vi "PH_PILS.Dialog EO.vi"() -> (0 "EO Comment":string)   [LabVIEW 2014, in "PH_PILS.lvlib"]
doc: "This VI creates the entry for the logbook in case of emergency off and writes it to the Logfile D:\\PCS_Logbook\\Log.txt."
uses:
  PH_PILS.lvlib
panel:
  in  "OK Button":bool
  in  "EO Comment":string
  # "Please enter a comment to explain the Emergency Off!"
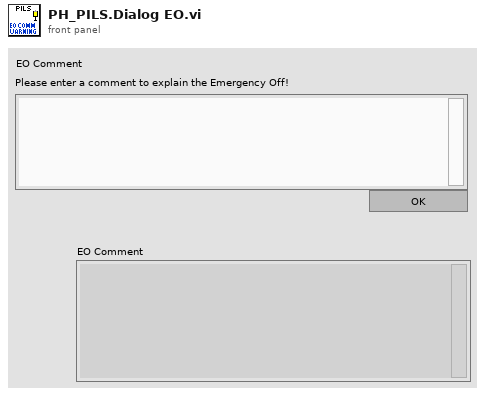
[diagram p1: front panel]
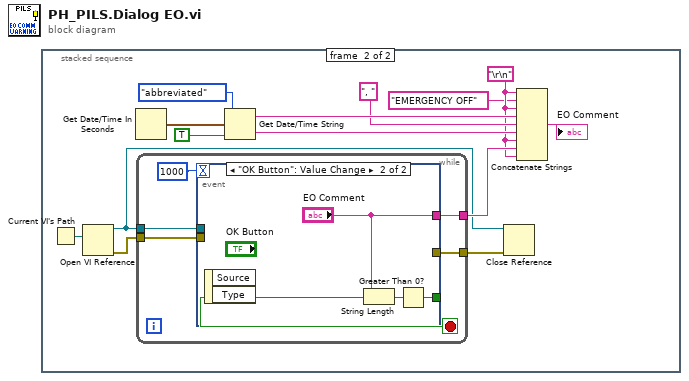
[diagram p0: block diagram]
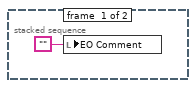
[diagram p2: hidden frame]
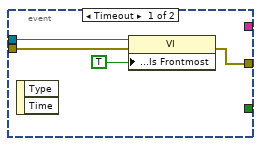
[diagram p3: hidden frame]
diagram:
  n1 = stacked-sequence {
    frame #0 {
      n2 = local write "EO Comment"("") -> ()
    }
    frame #1 {
      w3 = "\r\n"
      n3 = Current VI's Path() -> (path=w7:path)
      n4 = Open VI Reference(vi path=w7) -> (vi reference=w4:refnum<vi>, error out=w6:errorcluster)  [unwired: 5 in]
      n5 = Get Date/Time In Seconds() -> (seconds since 1Jan1904=w14:timestamp)
      n6 = while {
        tunnel: [w20] -> w9
        tunnel: w4 -> [w18]
        tunnel: w6 -> [w17]
        tunnel: [w16] -> w5
        stop <- w21 stop-if-true
        n7 = event shown="[1] \"OK Button\": Value Change" {
          selector: _ -> [_ _]
          dyn-events: _ -> [_ _]
          timeout: 1000 -> [_ _]
          tunnel: [_ w26] -> w21
          tunnel: [_ "EO Comment"] -> w20
          tunnel: w18 -> [w25 _]
          tunnel: w17 -> [w24 _]
          tunnel: [w22 _] -> w16
          event Timeout {
            n8 = event-data() -> ()  [unwired: 1 in, 2 out]
            n9 = property class="VI"(reference=w25, error in=w24, "Front Panel Window:Is Frontmost"=TRUE) -> (error out=w22:errorcluster)  [unwired: 1 out]
          }
          event "OK Button": Value Change {
            n10 = event-data() -> ()  [unwired: 1 in, 2 out]
            n11 = String Length(string="EO Comment") -> (length=w27:i32)
            n12 = Greater Than 0?(x=w27) -> (x > 0?=w26:bool)
          }
        }
      }
      n13 = Get Date/Time String(date format (0)=enum16{"short", "long", "abbreviated"}."abbreviated", seconds (now)=w14, want seconds? (F)=TRUE) -> (date string=w12:string, time string=w11:string)
      n14 = Close Reference(reference=w4, error in (no error)=w5) -> ()  [unwired: 1 out]
      n15 = Concatenate Strings(w3, "EMERGENCY OFF" ("string"), w3, w12, ", ", w11, w3, w9, w3) -> (→"EO Comment":string)
    }
  }
